vi "Prova Termica.vi"(6 "scale res":u16[](array[numeric]), 7 "Tipo motore pompa":enum16{"Monofase", "Trifase"}(ring), 8 "Solo acquisizione?":bool=TRUE, 9 "Manuale F\\auto T":bool=TRUE, 10 "Status":refnum<vi>, 11 "input cluster":T1={"Scelta wattmetro"={"Wattmetro"=enum."No Selection"}, "SET RPM"=0.0, "SET TEMP"=0.0, "Array banchi"=[{"Nome"="Elettropompa", "Tors. scala1"=0, "Tors. scala2"=0, "rpm"=0, "TAMB"=0, "Indici Temperature"=[0, 1], "Indice freno"=1, "alimentatore trifase"=0, "alimentatore monofase"=0, "alimentatore dc arm"=0, "alimentatore dc ecc"=0, "alimentatore dc mp"=0}, {"Nome"="Sommersa", "Tors. scala1"=0, "Tors. scala2"=0, "rpm"=0, "TAMB"=1, "Indici Temperature"=[0, 1], "Indice freno"=0, "alimentatore trifase"=0, "alimentatore monofase"=0, "alimentatore dc arm"=0, "alimentatore dc ecc"=0, "alimentatore dc mp"=0}], "Array valvole linee avvio/fermata"=[], "banco selezionato"=0, "Nomi valvole prop sistema"=[], "canale-- sensore"=[], "Attriti B1"=[], "Attriti B2"=[], "Collegamento elettrico"={"ALIMENTAZIONE ELETTRICA"=enum."AC MONOFASE", "ID"=0, "#rami freddo\\eq term resmeter"=0, "#rami riscaldamento resmeter"=0, "#rami freddo\\eq term resistomat"=0, "#rami riscaldamento resistomat"=0, "CALCOLI"=enum."AC TRIFASE"}, "lingua"=0, "Costanti collaudo"={"P [bar]"=0.0, "T amb. [°C]"=0.0, "Umidità [%]"=0.0, "T acqua [°C] 2"=0.0}, "OPZIONI MISURE RES"={"MISURA A FREDDO"=enum."RESISTOMAT", "MISURA EQ. TERMICO"=enum."RESISTOMAT", "MISURA DT PROVA IN CORSO"=enum."RESISTOMAT - CON FERMATE", "MISURE PRIMA E DOPO"=enum."RESISTOMAT", "STRUMENTI PRESENTI"=enum."NESSUNO"}, "Dati targa motore"={"Vnom"=0.0, "Fnom"=0.0, "Inom"=0.0, "Cnom"=0.0, "Npoli"=0.0, "Scorta 1"=0.0, "Scorta 2"=0.0, "Scorta 3"=0.0}}) -> ()   [LabVIEW 2019]
uses:
  TypeDef/ClusterRes.ctl
  Global settings termica.vi
  TypeDef/WT SELECTION.ctl
  TypeDef/Definizione linea.ctl
  TypeDef/Cluster INFO.ctl
  TypeDef/Collegamenti_elettrici.ctl
  TypeDef/Control Calcoli.ctl
panel:
  out "acq in corso":bool=TRUE
  out "Fermata":bool caption="Time has Elapsed"
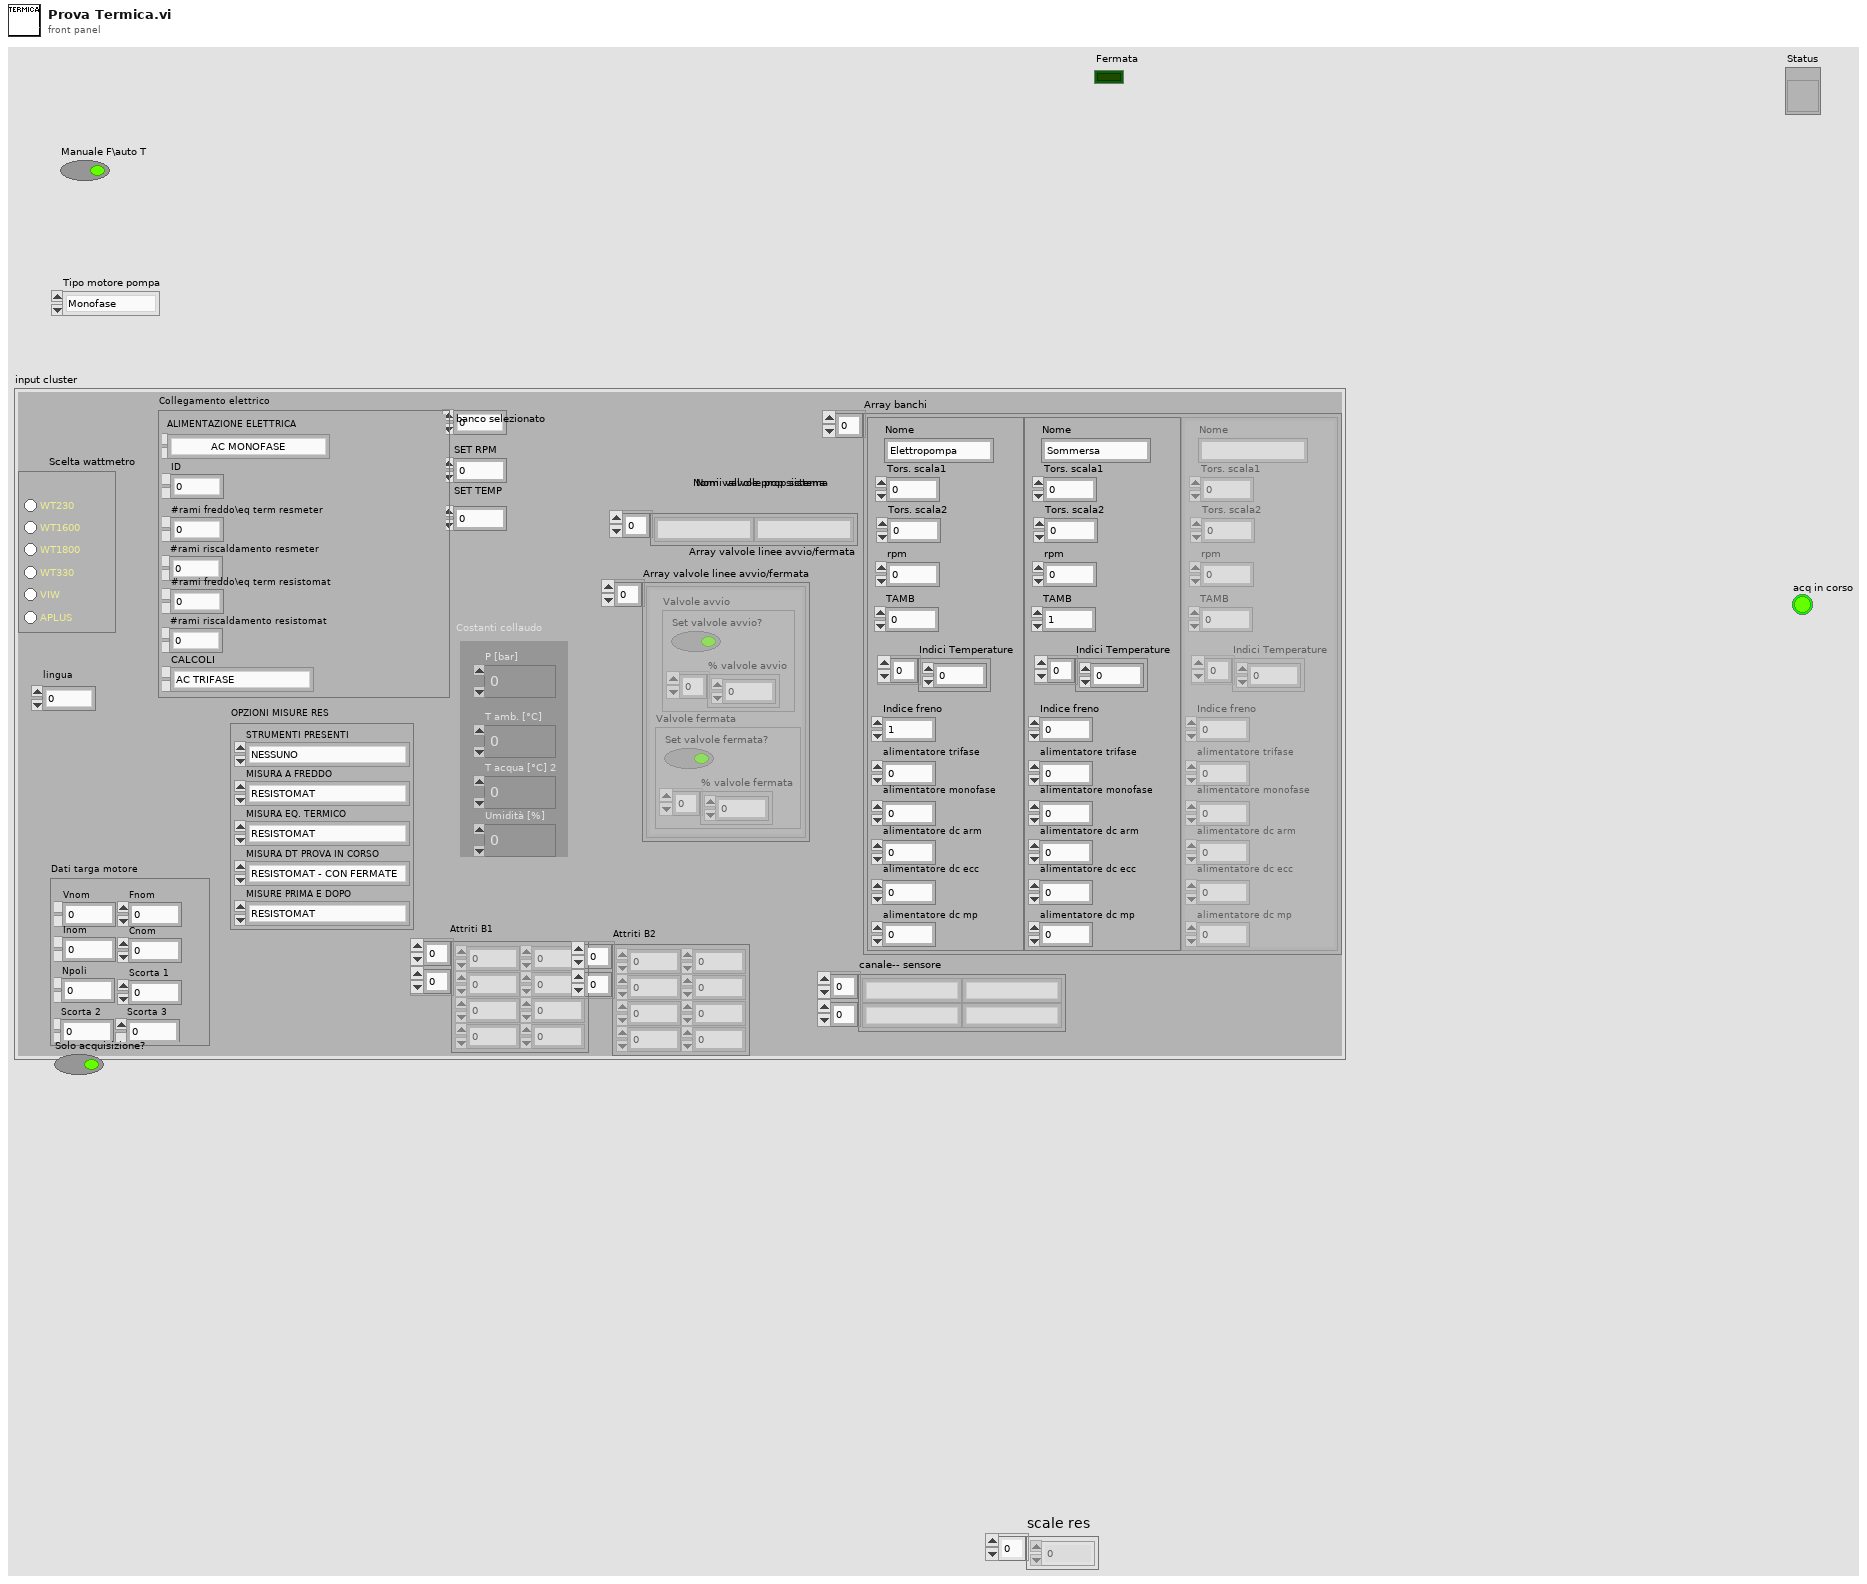
[diagram p1: front panel]
types:
  T1 = typedef "Cluster INFO.ctl" = cluster{"Scelta wattmetro":cluster{"Wattmetro":T2}, "SET RPM":dbl, "SET TEMP":dbl, "Array banchi":T3[], "Array valvole linee avvio/fermata":cluster{"Valvole avvio":cluster{"Set valvole avvio?":bool, "% valvole avvio":dbl[]}, "Valvole fermata":cluster{"Set valvole fermata?":bool, "% valvole fermata":dbl[]}}[], "banco selezionato":i8, "Nomi valvole prop sistema":string[], "canale-- sensore":string[][], "Attriti B1":dbl[][], "Attriti B2":dbl[][], "Collegamento elettrico":cluster{"ALIMENTAZIONE ELETTRICA":T4, "ID":i16, "#rami freddo\\eq term resmeter":i16, "#rami riscaldamento resmeter":i16, "#rami freddo\\eq term resistomat":i16, "#rami riscaldamento resistomat":i16, "CALCOLI":T5}, "lingua":i16, "Costanti collaudo":cluster{"P [bar]":dbl, "T amb. [°C]":dbl, "Umidità [%]":dbl, "T acqua [°C] 2":dbl}, "OPZIONI MISURE RES":cluster{"MISURA A FREDDO":enum16{"NESSUNO", "RESISTOMAT", "RES METER", "ENTRAMBI"}, "MISURA EQ. TERMICO":enum16{"NESSUNO", "RESISTOMAT", "RES METER", "ENTRAMBI"}, "MISURA DT PROVA IN CORSO":enum16{"NESSUNO", "RESISTOMAT - CON FERMATE", "RES METER - CON FERMATE", "RES METER - CONTINUO"}, "MISURE PRIMA E DOPO":enum16{"NESSUNO", "RESISTOMAT", "RES METER"}, "STRUMENTI PRESENTI":enum16{"NESSUNO", "RESISTOMAT", "RES METER", "ENTRAMBI"}}, "Dati targa motore":cluster{"Vnom":dbl, "Fnom":dbl, "Inom":dbl, "Cnom":dbl, "Npoli":dbl, "Scorta 1":dbl, "Scorta 2":dbl, "Scorta 3":dbl}}
  T2 = typedef "WT SELECTION.ctl" = enum32{"No Selection", "WT230", "WT1600", "WT1800", "WT330", "VIW", "APLUS"}
  T3 = typedef "Definizione linea.ctl" = cluster{"Nome":string, "Tors. scala1":i32, "Tors. scala2":i32, "rpm":i32, "TAMB":i32, "Indici Temperature":i16[], "Indice freno":i16, "alimentatore trifase":i16, "alimentatore monofase":i16, "alimentatore dc arm":i16, "alimentatore dc ecc":i16, "alimentatore dc mp":i16}
  T4 = typedef "Collegamenti_elettrici.ctl" = enum16{"AC TRIFASE", "AC TRIFASE + FRENO", "AC MONOFASE", "DC CON ECCITAZIONE", "DC CON ECCITAZIONE + FRENO", "DC NO ECCITAZIONE", "DC NO ECCITAZIONE + FRENO", "FRENO TRASC + AFE", "SOLO FRENO", "CARICO RESISTIVO", "GENERICO", "SOLO ACQUISITORE", "SCORTA 4", "SCORTA 5", "SCORTA 6"}
  T5 = typedef "Control Calcoli.ctl" = enum16{"AC TRIFASE", "AC MONOFASE", "DC ECCITAZIONE", "DC NO ECCITAZIONE", "POMPA TRIFASE", "POMPA MONOFASE", "GENERICO", "TRASFORMATORE", "ALTERNATORE TRASCINATO", "GRUPPO ELETTROGENO"}
  T6 = cluster{"Valvole avvio":cluster{"Set valvole avvio?":bool, "% valvole avvio":dbl[]}, "Valvole fermata":cluster{"Set valvole fermata?":bool, "% valvole fermata":dbl[]}}[]
  T7 = cluster{"Valvole avvio":cluster{"Set valvole avvio?":bool, "% valvole avvio":dbl[]}, "Valvole fermata":cluster{"Set valvole fermata?":bool, "% valvole fermata":dbl[]}}
  T8 = cluster{"Set valvole avvio?":bool, "% valvole avvio":dbl[]}
  T9 = cluster{"Set valvole fermata?":bool, "% valvole fermata":dbl[]}
  T10 = cluster{"Array of elements":cluster{"String":string, "variant":variant}[], "Single element":cluster{"String":string, "variant":variant}, "enque at\nopposite end (F)":bool, "no replications (F)":bool}
  T11 = typedef "ClusterRes.ctl" = cluster{"Res Ch1":dbl, "Res Ch2":dbl, "Res Ch3":dbl, "Tamb":dbl}
  T12 = typedef "Cluster termica.ctl" = cluster{"Tipo di servizio":u16, "s1":cluster{"Intervallo fermate":dbl}, "s3":cluster{"Tempo a carico":dbl, "Tempo a riposo":dbl}, "Tempo prova max":dbl, "Tempo acq auto":dbl, "Escludi mis res se stop":bool}
  T13 = cluster{"Tempo a carico":dbl, "Tempo a riposo":dbl}
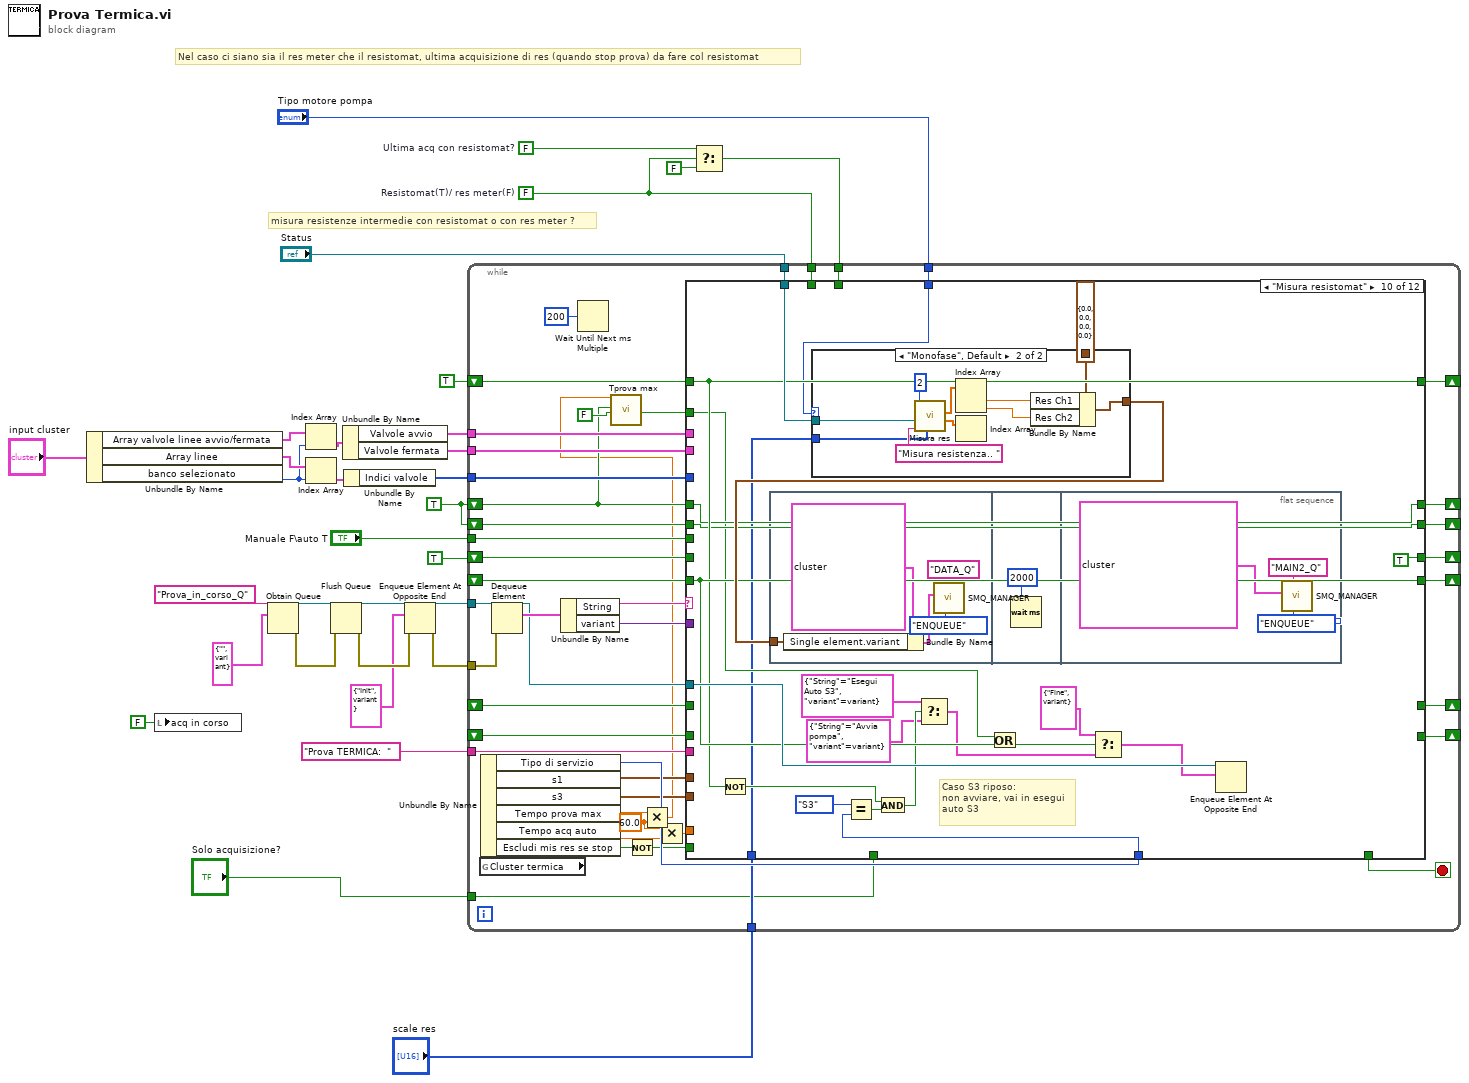
[diagram p0: block diagram]
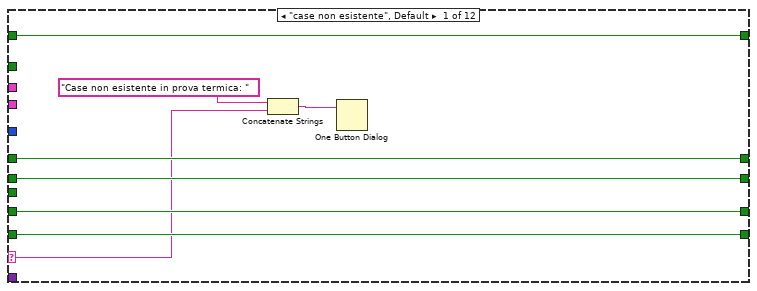
[diagram p2: hidden frame]
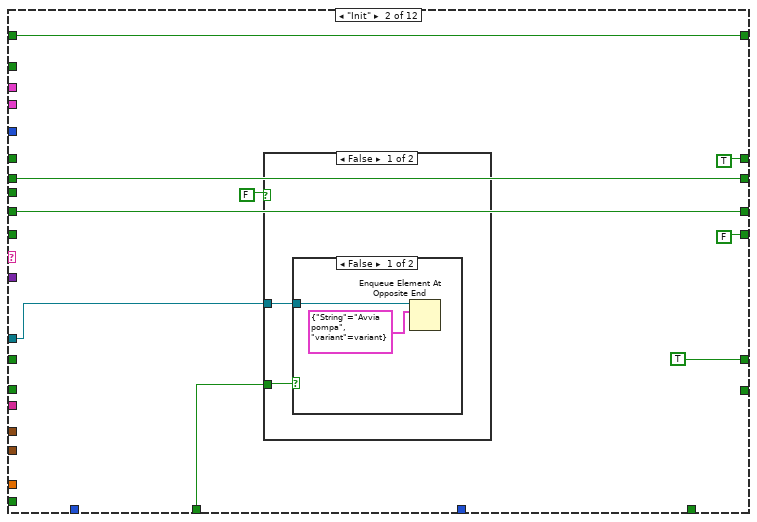
[diagram p3: hidden frame]
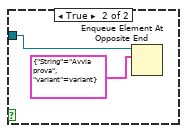
[diagram p4: hidden frame]
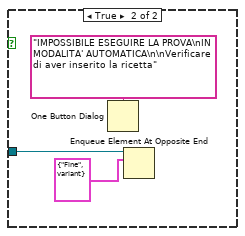
[diagram p5: hidden frame]
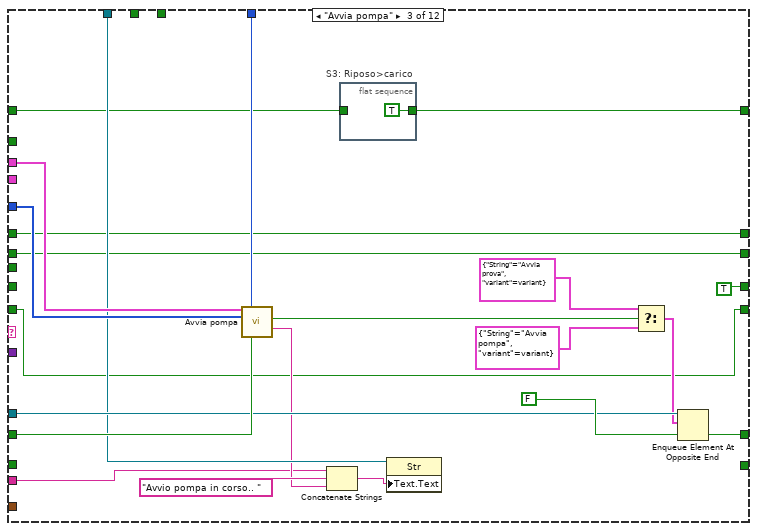
[diagram p6: hidden frame]
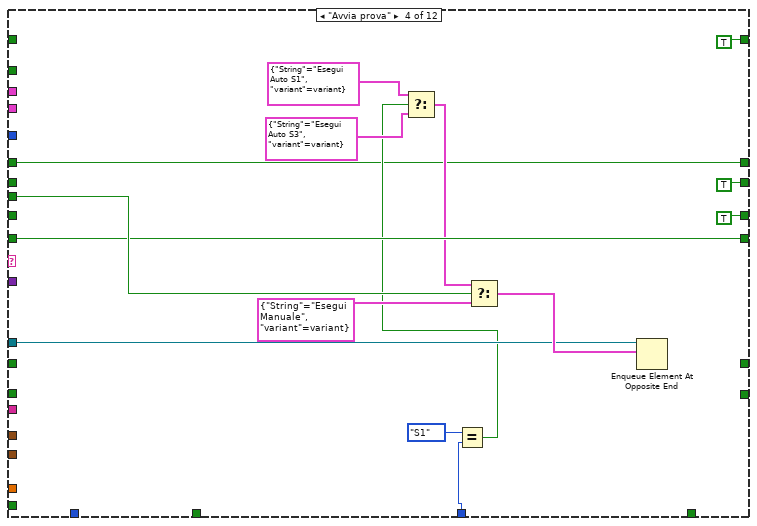
[diagram p7: hidden frame]
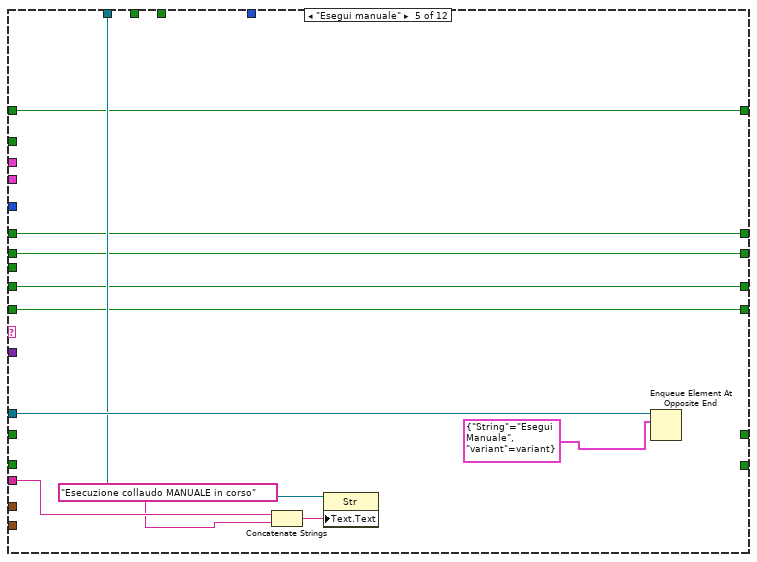
[diagram p8: hidden frame]
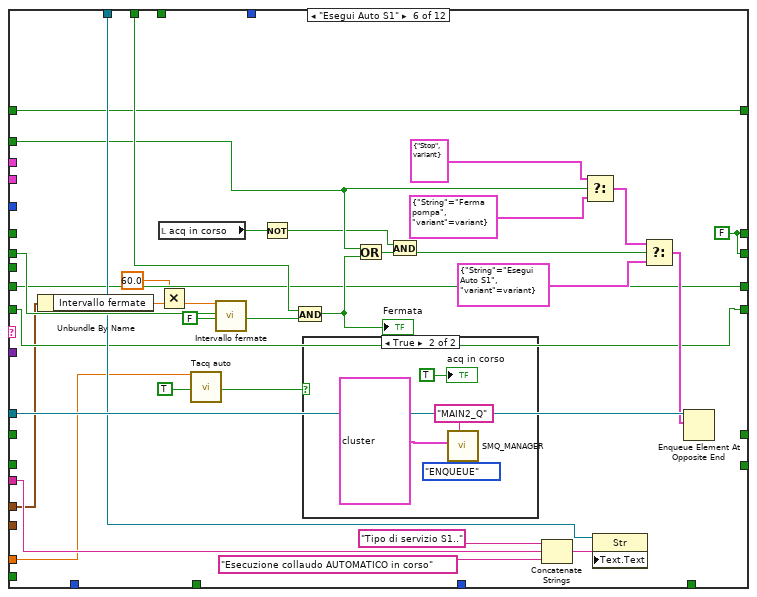
[diagram p9: hidden frame]
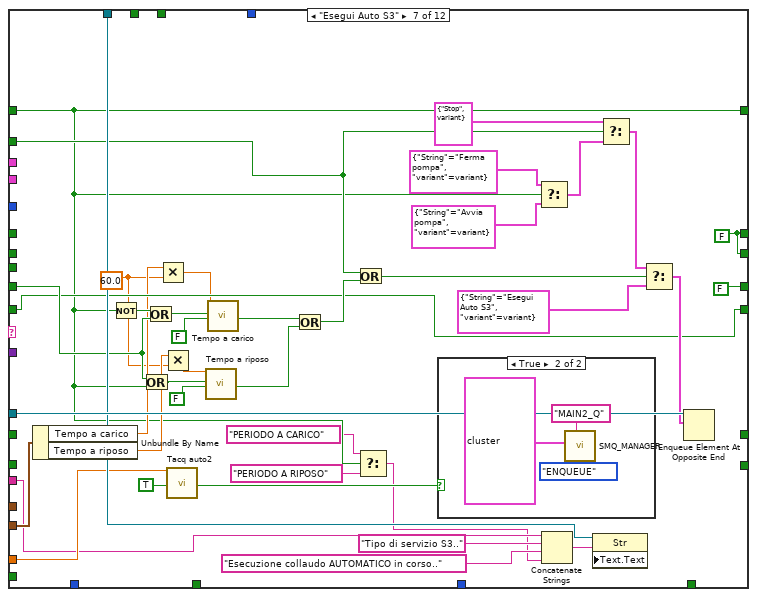
[diagram p11: hidden frame]
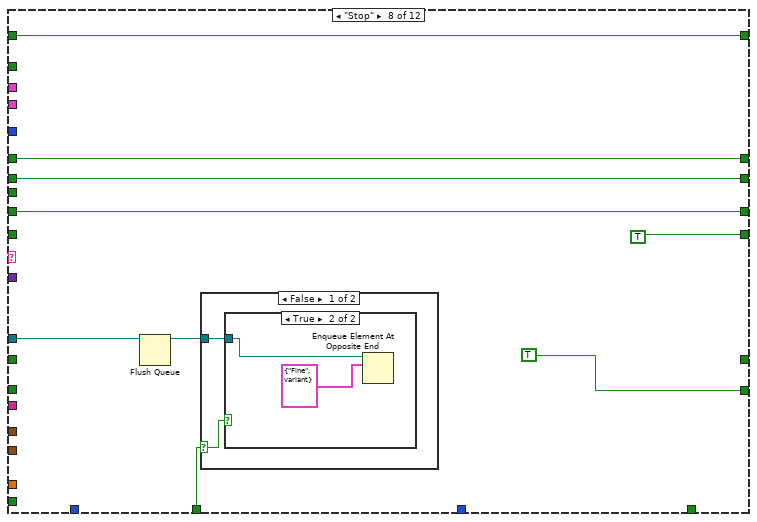
[diagram p13: hidden frame]
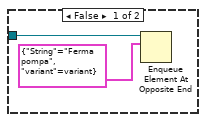
[diagram p14: hidden frame]
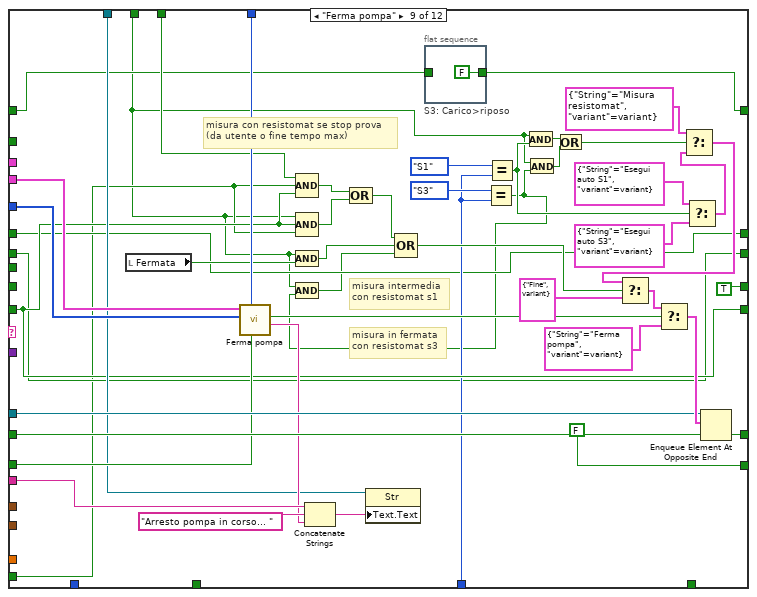
[diagram p16: hidden frame]
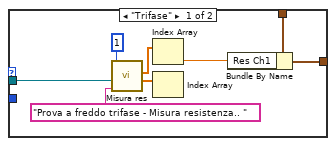
[diagram p17: hidden frame]
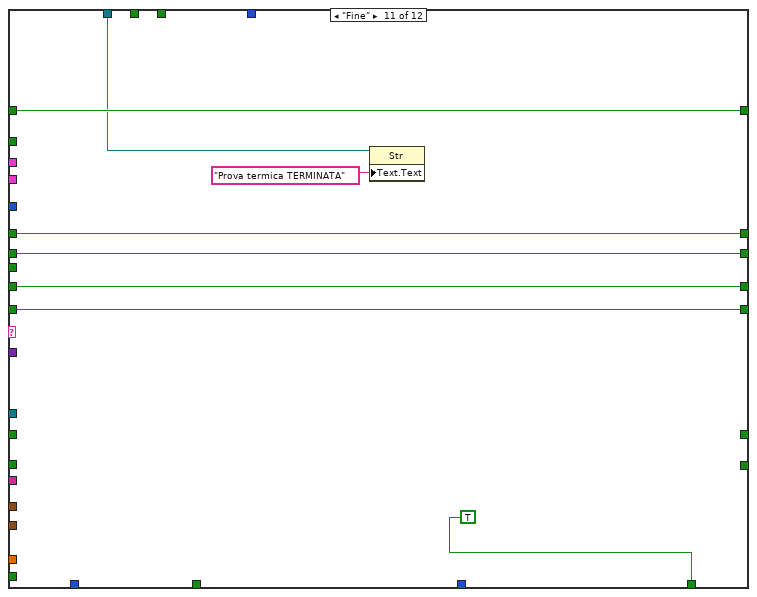
[diagram p18: hidden frame]
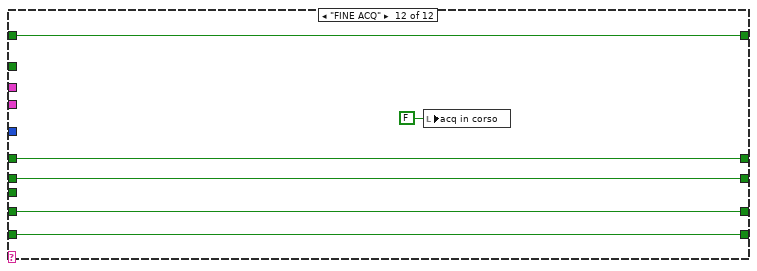
[diagram p19: hidden frame]
diagram:
  w8 = FALSE  # Ultima acq con resistomat?
  w11 = TRUE
  w10 = FALSE  # Resistomat(T)/ res meter(F)
  # "misura resistenze intermedie con resistomat o con res meter ?"
  # "Nel caso ci siano sia il res meter che il resistomat, ultima acquisizione di res (quando stop prova) da fare col resistomat"
  n1 = Unbundle By Name("input cluster") -> ("Array valvole linee avvio/fermata"=w20:T6, "Array linee"=w22:T3[], "banco selezionato"=w19:i8)
  n2 = local write "acq in corso"(FALSE ("acq in corso")) -> ()
  n3 = Obtain Queue(name (unnamed)="Prova_in_corso_Q" ("Queue Name"), element data type=cluster{"String":string, "variant":variant} {"String"="", "variant"=variant} ("element")) -> (queue out=w27:refnum<queue>, error out=w26:errorcluster)  [unwired: 3 in, 1 out]
  n4 = Index Array(array=w20, index=w19) -> (element=w18:T7)
  n5 = Index Array(array=w22, index=w19) -> (element=w21:T3)
  n6 = Flush Queue(queue=w27, error in (no error)=w26) -> (queue out=w30:refnum<queue>, error out=w29:errorcluster)  [unwired: 1 out]
  n7 = Unbundle By Name(w18) -> ("Valvole avvio"=w16:T8, "Valvole fermata"=w15:T9)
  n8 = Unbundle By Name(w21) -> ("Indici valvole"=w14:i16[])
  n9 = Enqueue Element At Opposite End(queue=w30, element=cluster{"String":string, "variant":variant} {"String"="Init", "variant"=variant}, error in (no error)=w29) -> (queue out=w32:refnum<queue>, error out=w31:errorcluster)  [unwired: 1 in, 1 out]
  n10 = Select(t=w8, s=w10, f=FALSE) -> (s? t:f=w9:bool)
  n11 = while {
    tunnel: w32 -> [w78]
    tunnel: w31 -> [w77]
    tunnel: "Manuale F\\auto T" -> [w73]
    shift-right: [w71] -> _
    shift-left: _ -> [w70]
    tunnel: w16 -> [w69]
    tunnel: "Tipo motore pompa" -> [w68]
    tunnel: w15 -> [w67]
    shift-right: [w66] -> _
    shift-left: _ -> [w65]
    tunnel: w14 -> [w64]
    tunnel: "Status" -> [w63]
    tunnel: "Prova TERMICA:  " ("Text.Text") -> [w61]
    tunnel: w10 -> [w57]
    shift-right: [w60] -> _
    shift-left: w11 -> [w36]
    shift-right: [w58] -> _
    shift-left: w11 -> [w59]
    shift-right: [w56] -> _
    shift-left: _ -> [w55]
    tunnel: w9 -> [w54]
    shift-right: [w52] -> _
    shift-left: TRUE -> [w53]
    shift-right: [w50] -> _
    shift-left: TRUE -> [w51]
    tunnel: "scale res" -> [w34]
    tunnel: "Solo acquisizione?" -> [w33]
    stop <- w62 stop-if-true
    w40 = 60.0 ("y")
    n12 = global read "Global settings termica.vi" "Cluster termica"() -> (w49:T12)
    n13 = Unbundle By Name(w49) -> ("Tipo di servizio"=w48:u16, "s1"=w47:cluster{"Intervallo fermate":dbl}, "s3"=w44:T13, "Tempo prova max"=w46:dbl, "Tempo acq auto"=w45:dbl, "Escludi mis res se stop"=w43:bool)
    n14 = Dequeue Element(queue=w78, error in (no error)=w77) -> (queue out=w72:refnum<queue>, element=w76:cluster{"String":string, "variant":variant})  [unwired: 1 in, 2 out]
    n15 = Unbundle By Name(w76) -> ("String"=w75:string, "variant"=w74:variant)
    n16 = Wait Until Next ms Multiple(millisecond multiple=u32 200) -> ()  [unwired: 1 out]
    n17 = Not(x=w43) -> (.not. x?=w42:bool)
    n18 = Multiply(x=w46, y=w40) -> (x*y=w35:dbl)
    n19 = call "Tprova max"("Time Target (s)"=w35, "Reset"=w36, "Auto Reset"=FALSE ("Reset")) -> ("Time has Elapsed"=w37:bool)  [unwired: 9 in, 7 out]
    n20 = Multiply(x=w40, y=w45) -> (x*y=w41:dbl)
    n21 = case shown="\"Misura resistomat\"" w75 {
      selector: w75 -> [w81 _ _ _ _ _ _ _ _ _ _ _]
      tunnel: w74 -> [_ _ _ _ _ _ _ _ _ _ _ _]
      tunnel: w73 -> [_ _ _ w138 _ _ _ _ _ _ _ _]
      tunnel: w72 -> [_ w95 w123 w139 w151 w178 w225 w240 w286 w313 _ _]
      tunnel: [_ TRUE FALSE _ _ _ _ _ w290 _ _ _] -> w71
      tunnel: w70 -> [_ _ w125 _ _ _ _ _ w290 _ _ _]
      tunnel: w69 -> [_ _ w117 _ _ _ _ _ _ _ _ _]
      tunnel: w68 -> [_ _ w118 _ _ _ _ _ w291 w298 _ _]
      tunnel: w67 -> [_ _ _ _ _ _ _ _ w284 _ _ _]
      tunnel: [_ _ _ _ _ _ _ TRUE FALSE _ _ _] -> w66
      tunnel: w65 -> [_ _ _ _ _ _ _ _ w285 _ _ _]
      tunnel: w64 -> [_ _ w116 _ _ _ _ _ w283 _ _ _]
      tunnel: w63 -> [_ _ w115 _ w150 w165 w216 _ w278 w316 w345 _]
      tunnel: [_ _ _ _ _ _ _ _ _ _ TRUE _] -> w62
      tunnel: w61 -> [_ _ w111 _ w149 w182 w194 _ w281 _ _ _]
      tunnel: w36 -> [w86 _ w107 w127 w144 _ _ w235 w254 w300 w348 w357]
      tunnel: [w86 TRUE w107 w127 w144 w179 w226 w235 w254 w300 w348 w357] -> w60
      tunnel: w59 -> [w85 w92 w106 _ w143 w181 _ w234 w253 w299 w347 w356]
      tunnel: [w85 w92 w106 TRUE w143 w179 w226 w234 w253 w299 w347 w356] -> w58
      tunnel: w57 -> [_ _ _ _ _ w173 _ _ w249 _ _ _]
      tunnel: [w84 FALSE w108 w137 w145 w163 w204 TRUE w268 w311 w349 w355] -> w56
      tunnel: w55 -> [w84 _ w108 w137 w145 w163 w204 _ w268 w311 w349 w355]
      tunnel: w54 -> [_ _ _ _ _ _ _ _ w269 _ _ _]
      tunnel: w53 -> [w83 w93 w110 _ w142 w162 w192 w233 w261 w306 w346 w354]
      tunnel: [w83 w93 w109 TRUE w142 w162 w192 w233 w260 w306 w346 w354] -> w52
      tunnel: w51 -> [w82 w91 _ _ w146 w164 w206 w236 _ _ w350 w353]
      tunnel: [w82 w91 TRUE TRUE w146 w164 FALSE w236 TRUE TRUE w350 w353] -> w50
      tunnel: w48 -> [_ _ _ w134 _ _ _ _ w257 w307 _ _]
      tunnel: w47 -> [_ _ _ _ _ w161 _ _ _ _ _ _]
      tunnel: w41 -> [_ _ _ _ _ w159 w203 _ _ _ _ _]
      tunnel: w44 -> [_ _ _ _ _ _ w202 _ _ _ _ _]
      tunnel: w42 -> [_ _ _ _ _ _ _ _ w252 _ _ _]
      tunnel: w37 -> [_ _ _ _ _ w156 w196 _ _ w296 _ _]
      tunnel: w34 -> [_ _ _ _ _ _ _ _ _ w294 _ _]
      tunnel: w33 -> [_ w87 _ _ _ _ _ w232 _ _ _ _]
      frame "case non esistente", Default {
        n22 = Concatenate Strings("Case non esistente in prova termica: " ("string"), w81) -> (w80:string)
        n23 = One Button Dialog(message=w80) -> ()  [unwired: 1 in, 1 out]
      }
      frame "Init" {
        n24 = case shown="False" FALSE {
          tunnel: w95 -> [w97 w103]
          tunnel: w87 -> [w96 _]
          frame False {
            n25 = case shown="False" w96 {
              tunnel: w97 -> [w98 w100]
              frame False {
                n26 = Enqueue Element At Opposite End(queue=w98, element=cluster{"String":string, "variant":variant} {"String"="Avvia pompa", "variant"=variant}) -> ()  [unwired: 2 in, 3 out]
              }
              frame True {
                n27 = Enqueue Element At Opposite End(queue=w100, element=cluster{"String":string, "variant":variant} {"String"="Avvia prova", "variant"=variant}) -> ()  [unwired: 2 in, 3 out]
              }
            }
          }
          frame True {
            n28 = One Button Dialog(message="IMPOSSIBILE ESEGUIRE LA PROVA\nIN MODALITA' AUTOMATICA\n\nVerificare di aver inserito la ricetta") -> ()  [unwired: 1 in, 1 out]
            n29 = Enqueue Element At Opposite End(queue=w103, element=cluster{"String":string, "variant":variant} {"String"="Fine", "variant"=variant}) -> ()  [unwired: 2 in, 3 out]
          }
        }
      }
      frame "Avvia pompa" {
        n30 = call "Avvia pompa.vi"("Valvole avvio"=w117, "Tipo motore pompa"=w118, "Indici valvole linea"=w116, "Reset avvio"=w125) -> ("Fine Avvio"=w122:bool, "stato"=w112:string)  [unwired: 10 in]
        n31 = Concatenate Strings(w111, "Avvio pompa in corso.. " ("Text.Text"), w112) -> (w113:string)
        n32 = flat-sequence "S3: Riposo>carico" {
          tunnel: w110 -> [_]
          tunnel: [TRUE] -> w109
          frame #0 {
          }
        }
        n33 = property class="Str"(reference=w115, "Text.Text"=w113) -> ()  [unwired: 1 in, 2 out]
        n34 = Select(t=cluster{"String":string, "variant":variant} {"String"="Avvia prova", "variant"=variant} ("element"), s=w122, f=cluster{"String":string, "variant":variant} {"String"="Avvia pompa", "variant"=variant} ("element")) -> (s? t:f=w120:cluster{"String":string, "variant":variant})
        n35 = Enqueue Element At Opposite End(queue=w123, element=w120) -> ()  [unwired: 2 in, 3 out]
      }
      frame "Avvia prova" {
        n36 = Equal?(x=enum16{"S1", "S3"}."S1", y=w134) -> (x = y?=w132:bool)
        n37 = Select(t=cluster{"String":string, "variant":variant} {"String"="Esegui Auto S1", "variant"=variant} ("element"), s=w132, f=cluster{"String":string, "variant":variant} {"String"="Esegui Auto S3", "variant"=variant} ("element")) -> (s? t:f=w131:cluster{"String":string, "variant":variant})
        n38 = Select(t=w131, s=w138, f=cluster{"String":string, "variant":variant} {"String"="Esegui Manuale", "variant"=variant} ("element")) -> (s? t:f=w140:cluster{"String":string, "variant":variant})
        n39 = Enqueue Element At Opposite End(queue=w139, element=w140) -> ()  [unwired: 2 in, 3 out]
      }
      frame "Esegui manuale" {
        n40 = Concatenate Strings(w149, "Esecuzione collaudo MANUALE in corso" ("string")) -> (w148:string)
        n41 = property class="Str"(reference=w150, "Text.Text"=w148) -> ()  [unwired: 1 in, 2 out]
        n42 = Enqueue Element At Opposite End(queue=w151, element=cluster{"String":string, "variant":variant} {"String"="Esegui Manuale", "variant"=variant}) -> ()  [unwired: 2 in, 3 out]
      }
      frame "Esegui Auto S1" {
        w179 = FALSE
        n43 = Unbundle By Name(w161) -> ("Intervallo fermate"=w160:dbl)
        n44 = local read "acq in corso"() -> (w155:bool)
        n45 = Multiply(x=60.0, y=w160) -> (x*y=w158:dbl)
        n46 = call "Tacq auto"("Time Target (s)"=w159, "Auto Reset"=TRUE) -> ("Time has Elapsed"=w168:bool)  [unwired: 10 in, 7 out]
        n47 = call "Intervallo fermate"("Time Target (s)"=w158, "Reset"=w181, "Auto Reset"=FALSE) -> ("Time has Elapsed"=w175:bool)  [unwired: 9 in, 7 out]
        n48 = Not(x=w155) -> (.not. x?=w153:bool)
        n49 = And(x=w173, y=w175) -> (x .and. y?=w172:bool)
        "Fermata" <- w172
        n50 = case shown="True" w168 {
          frame False {
          }
          frame True {
            n51 = call <userlib>:"SMQ_MANAGER.vi"("Function"=enum16{"INITIALIZE", "ENQUEUE", "STOP ALL"}."ENQUEUE", "Queue name"="MAIN2_Q", "Enqueue cluster"=T10 {"Array of elements"=[], "Single element"={"String"="AQ AUTO", "variant"=variant}, "enque at\nopposite end (F)"=FALSE, "no replications (F)"=FALSE}) -> ()  [unwired: 8 in, 1 out]
            "acq in corso" <- TRUE
          }
        }
        n52 = Or(x=w156, y=w172) -> (x .or. y?=w174:bool)
        n53 = And(x=w153, y=w174) -> (x .and. y?=w154:bool)
        n54 = Concatenate Strings("Tipo di servizio S1.." ("string"), w182, "Esecuzione collaudo AUTOMATICO in corso" ("string")) -> (w184:string)
        n55 = Select(t=cluster{"String":string, "variant":variant} {"String"="Stop", "variant"=variant} ("element"), s=w156, f=cluster{"String":string, "variant":variant} {"String"="Ferma pompa", "variant"=variant} ("element")) -> (s? t:f=w170:cluster{"String":string, "variant":variant})
        n56 = property class="Str"(reference=w165, "Text.Text"=w184) -> ()  [unwired: 1 in, 2 out]
        n57 = Select(t=w170, s=w154, f=cluster{"String":string, "variant":variant} {"String"="Esegui Auto S1", "variant"=variant} ("element")) -> (s? t:f=w176:cluster{"String":string, "variant":variant})
        n58 = Enqueue Element At Opposite End(queue=w178, element=w176) -> ()  [unwired: 2 in, 3 out]
      }
      frame "Esegui Auto S3" {
        w197 = 60.0 ("y")
        w226 = FALSE
        n59 = Unbundle By Name(w202) -> ("Tempo a carico"=w201:dbl, "Tempo a riposo"=w200:dbl)
        n60 = Not(x=w192) -> (.not. x?=w210:bool)
        n61 = Or(x=w206, y=w192) -> (x .or. y?=w207:bool)
        n62 = Or(x=w210, y=w206) -> (x .or. y?=w208:bool)
        n63 = Multiply(x=w201, y=w197) -> (x*y=w199:dbl)
        n64 = Multiply(x=w200, y=w197) -> (x*y=w198:dbl)
        n65 = call "Tacq auto2"("Time Target (s)"=w203, "Auto Reset"=TRUE) -> ("Time has Elapsed"=w218:bool)  [unwired: 10 in, 7 out]
        n66 = call "Tempo a riposo"("Time Target (s)"=w198, "Reset"=w207, "Auto Reset"=FALSE) -> ("Time has Elapsed"=w214:bool)  [unwired: 9 in, 7 out]
        n67 = call "Tempo a carico"("Time Target (s)"=w199, "Reset"=w208, "Auto Reset"=FALSE) -> ("Time has Elapsed"=w209:bool)  [unwired: 9 in, 7 out]
        n68 = Or(x=w209, y=w214) -> (x .or. y?=w221:bool)
        n69 = Or(x=w196, y=w221) -> (x .or. y?=w222:bool)
        n70 = Select(t="PERIODO A CARICO" ("string"), s=w192, f="PERIODO A RIPOSO" ("string")) -> (s? t:f=w189:string)
        n71 = case shown="True" w218 {
          frame False {
          }
          frame True {
            n72 = call <userlib>:"SMQ_MANAGER.vi"("Function"=enum16{"INITIALIZE", "ENQUEUE", "STOP ALL"}."ENQUEUE", "Queue name"="MAIN2_Q", "Enqueue cluster"=T10 {"Array of elements"=[], "Single element"={"String"="AQ AUTO", "variant"=variant}, "enque at\nopposite end (F)"=FALSE, "no replications (F)"=FALSE}) -> ()  [unwired: 8 in, 1 out]
          }
        }
        n73 = Select(t=cluster{"String":string, "variant":variant} {"String"="Ferma pompa", "variant"=variant} ("element"), s=w192, f=cluster{"String":string, "variant":variant} {"String"="Avvia pompa", "variant"=variant} ("element")) -> (s? t:f=w212:cluster{"String":string, "variant":variant})
        n74 = Concatenate Strings(w194, "Tipo di servizio S3.." ("string"), "Esecuzione collaudo AUTOMATICO in corso.." ("string"), w189) -> (w228:string)
        n75 = property class="Str"(reference=w216, "Text.Text"=w228) -> ()  [unwired: 1 in, 2 out]
        n76 = Select(t=cluster{"String":string, "variant":variant} {"String"="Stop", "variant"=variant} ("element"), s=w196, f=w212) -> (s? t:f=w220:cluster{"String":string, "variant":variant})
        n77 = Select(t=w220, s=w222, f=cluster{"String":string, "variant":variant} {"String"="Esegui Auto S3", "variant"=variant} ("element")) -> (s? t:f=w223:cluster{"String":string, "variant":variant})
        n78 = Enqueue Element At Opposite End(queue=w225, element=w223) -> ()  [unwired: 2 in, 3 out]
      }
      frame "Stop" {
        n79 = Flush Queue(queue=w240) -> (queue out=w239:refnum<queue>)  [unwired: 1 in, 2 out]
        n80 = case shown="False" w232 {
          selector: w232 -> [w241 _]
          tunnel: w239 -> [w242 _]
          frame False {
            n81 = case shown="True" w241 {
              tunnel: w242 -> [w243 w245]
              frame False {
                n82 = Enqueue Element At Opposite End(queue=w243, element=cluster{"String":string, "variant":variant} {"String"="Ferma pompa", "variant"=variant}) -> ()  [unwired: 2 in, 3 out]
              }
              frame True {
                n83 = Enqueue Element At Opposite End(queue=w245, element=cluster{"String":string, "variant":variant} {"String"="Fine", "variant"=variant}) -> ()  [unwired: 2 in, 3 out]
              }
            }
          }
          frame True {
          }
        }
      }
      frame "Ferma pompa" {
        # "misura in fermata\ncon resistomat s3"
        # "misura con resistomat se stop prova\n(da utente o fine tempo max)"
        # "misura intermedia\ncon resistomat s1"
        n84 = local read "Fermata"() -> (w275:bool)
        n85 = call "Ferma pompa.vi"("Reset fermata"=w285, "Tipo motore pompa"=w291, "Indici valvole linea"=w283, "Valvole fermata"=w284) -> ("stato"=w279:string, "Fine Fermata"=w287:bool)  [unwired: 6 in]
        n86 = Compound Arithmetic op=AND(w269, w252, w268) -> (w270:bool)
        n87 = Compound Arithmetic op=AND(w249, w268, w252) -> (w272:bool)
        n88 = Compound Arithmetic op=AND(w249, w275) -> (w274:bool)
        n89 = Concatenate Strings(w281, "Arresto pompa in corso... " ("string"), w279) -> (w282:string)
        n90 = Compound Arithmetic op=OR(w270, w272) -> (w271:bool)
        n91 = property class="Str"(reference=w278, "Text.Text"=w282) -> ()  [unwired: 1 in, 2 out]
        n92 = flat-sequence "S3: Carico>riposo" {
          tunnel: w261 -> [_]
          tunnel: [FALSE] -> w260
          frame #0 {
          }
        }
        n93 = Equal?(x=enum16{"S1", "S3"}."S3", y=w257) -> (x = y?=w248:bool)
        n94 = Compound Arithmetic op=AND(w249, w248) -> (w250:bool)
        n95 = Compound Arithmetic op=OR(w271, w274, w250) -> (w273:bool)
        n96 = Equal?(x=enum16{"S1", "S3"}."S1", y=w257) -> (x = y?=w251:bool)
        n97 = And(x=w249, y=w251) -> (x .and. y?=w259:bool)
        n98 = And(x=w249, y=w248) -> (x .and. y?=w256:bool)
        n99 = Or(x=w259, y=w256) -> (x .or. y?=w255:bool)
        n100 = Select(t=cluster{"String":string, "variant":variant} {"String"="Esegui auto S1", "variant"=variant} ("element"), s=w251, f=cluster{"String":string, "variant":variant} {"String"="Esegui auto S3", "variant"=variant} ("element")) -> (s? t:f=w263:cluster{"String":string, "variant":variant})
        n101 = Select(t=cluster{"String":string, "variant":variant} {"String"="Misura resistomat", "variant"=variant} ("element"), s=w255, f=w263) -> (s? t:f=w262:cluster{"String":string, "variant":variant})
        n102 = Select(t=w262, s=w273, f=cluster{"String":string, "variant":variant} {"String"="Fine", "variant"=variant} ("element")) -> (s? t:f=w276:cluster{"String":string, "variant":variant})
        n103 = Select(t=w276, s=w287, f=cluster{"String":string, "variant":variant} {"String"="Ferma pompa", "variant"=variant} ("element")) -> (s? t:f=w288:cluster{"String":string, "variant":variant})
        n104 = Enqueue Element At Opposite End(queue=w286, element=w288) -> ()  [unwired: 2 in, 3 out]
      }
      frame "Misura resistomat" {
        # "Caso S3 riposo:\nnon avviare, vai in esegui\nauto S3"
        n105 = Not(x=w306) -> (.not. x?=w305:bool)
        n106 = flat-sequence {
          tunnel: w314 -> [w317]
          frame #0 {
            n107 = Bundle By Name(cluster=T10 {"Array of elements"=[], "Single element"={"String"="READ RESISTENZE", "variant"=variant}, "enque at\nopposite end (F)"=FALSE, "no replications (F)"=FALSE} ("Enqueue cluster"), "Single element.variant"=w317) -> (w318:T10)
            n108 = call <userlib>:"SMQ_MANAGER.vi"("Function"=enum16{"INITIALIZE", "ENQUEUE", "STOP ALL"}."ENQUEUE", "Queue name"="DATA_Q", "Enqueue cluster"=w318) -> ()  [unwired: 8 in, 1 out]
          }
          frame #1 {
            n109 = Wait (ms)(milliseconds to wait=u32 2000) -> ()  [unwired: 1 out]
          }
          frame #2 {
            n110 = call <userlib>:"SMQ_MANAGER.vi"("Function"=enum16{"INITIALIZE", "ENQUEUE", "STOP ALL"}."ENQUEUE", "Queue name"="MAIN2_Q", "Enqueue cluster"=T10 {"Array of elements"=[], "Single element"={"String"="ACQ CALDO RESISTOMAT", "variant"=variant}, "enque at\nopposite end (F)"=FALSE, "no replications (F)"=FALSE}) -> ()  [unwired: 8 in, 1 out]
          }
        }
        n111 = case shown="\"Monofase\", Default" w298 {
          tunnel: w316 -> [w329 w339]
          tunnel: T11 {"Res Ch1"=0.0, "Res Ch2"=0.0, "Res Ch3"=0.0, "Tamb"=0.0} ("Cluster Resistenze") -> [w328 w338]
          tunnel: [w326 w336] -> w314
          tunnel: w294 -> [_ w334]
          frame "Trifase" {
            n112 = call "Misura res.vi"("String"="Prova a freddo trifase - Misura resistenza.. ", "Status"=w329, "N°rami"=1) -> ("temperature amb"=w331:dbl[], "Valori res (ohm)"=w330:dbl[])  [unwired: 6 in, 1 out]
            n113 = Index Array(array=w330) -> (element=w327:dbl)  [unwired: 1 in]
            n114 = Index Array(array=w331) -> ()  [unwired: 1 in, 1 out]
            n115 = Bundle By Name(cluster=w328, "Res Ch1"=w327) -> (w326:T11)
          }
          frame "Monofase", Default {
            n116 = call "Misura res.vi"("Scala per ramo"=w334, "String"="Misura resistenza.. ", "Status"=w339, "N°rami"=2) -> ("temperature amb"=w341:dbl[], "Valori res (ohm)"=w340:dbl[])  [unwired: 5 in, 1 out]
            n117 = Index Array(array=w340) -> (element #1=w337:dbl, element #2=w335:dbl)  [unwired: 2 in]
            n118 = Index Array(array=w341) -> ()  [unwired: 1 in, 1 out]
            n119 = Bundle By Name(cluster=w338, "Res Ch1"=w337, "Res Ch2"=w335) -> (w336:T11)
          }
        }
        n120 = Equal?(x=enum16{"S1", "S3"}."S3", y=w307) -> (x = y?=w309:bool)
        n121 = And(x=w305, y=w309) -> (x .and. y?=w303:bool)
        n122 = Select(t=cluster{"String":string, "variant":variant} {"String"="Esegui Auto S3", "variant"=variant} ("f"), s=w303, f=cluster{"String":string, "variant":variant} {"String"="Avvia pompa", "variant"=variant} ("element")) -> (s? t:f=w304:cluster{"String":string, "variant":variant})
        n123 = Or(x=w296, y=w311) -> (x .or. y?=w297:bool)
        n124 = Select(t=cluster{"String":string, "variant":variant} {"String"="Fine", "variant"=variant} ("element"), s=w297, f=w304) -> (s? t:f=w312:cluster{"String":string, "variant":variant})
        n125 = Enqueue Element At Opposite End(queue=w313, element=w312) -> ()  [unwired: 2 in, 3 out]
      }
      frame "Fine" {
        n126 = property class="Str"(reference=w345, "Text.Text"="Prova termica TERMINATA") -> ()  [unwired: 1 in, 2 out]
      }
      frame "FINE ACQ" {
        n127 = local write "acq in corso"(FALSE ("acq in corso")) -> ()
      }
    }
  }
